vi "Parse Arguments.vi"(8 "error in (no error)":errorcluster, 9 "Args":string[](array[string]), 10 "Folder":path, 11 "UpdateAction in":refnum<class "UpdateAction.lvclass">) -> (0 "error out":errorcluster, 3 "UpdateAction out":refnum<class "UpdateAction.lvclass">)   [LabVIEW 2020, in "GPackTools.lvlib" / "UpdateAction.lvclass"]
uses:
  UpdateAction.lvclass
  UpdateAction.lvclass/UpdateAction.ctl
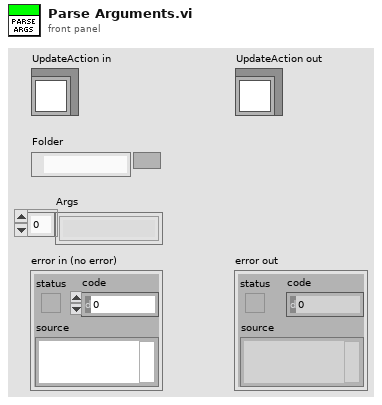
[diagram p1: front panel]
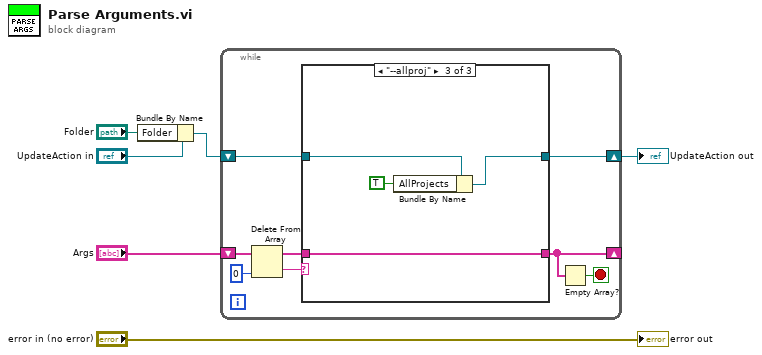
[diagram p0: block diagram]
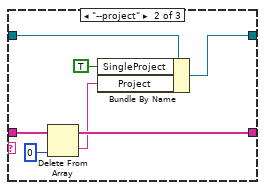
[diagram p3: hidden frame]
diagram:
  n1 = Bundle By Name(cluster="UpdateAction in", "Folder"="Folder") -> (w2:refnum<class "UpdateAction.lvclass">)
  n2 = while {
    shift-right: [w7] -> w3
    shift-left: w2 -> [w8]
    shift-right: [w10] -> _
    shift-left: "Args" -> [w14]
    stop <- w9 stop-if-true
    n3 = Delete From Array(array=w14, index=0) -> (deleted portion=w12:string, array with subset deleted=w11:string[])  [unwired: 1 in]
    n4 = case shown="\"--allproj\"" w12 {
      tunnel: w11 -> [w16 w22 w27]
      tunnel: [w16 w20 w27] -> w10
      tunnel: w8 -> [w15 w23 w26]
      tunnel: [w15 w19 w25] -> w7
      frame Default {
      }
      frame "--project" {
        n5 = Delete From Array(array=w22, index=0) -> (deleted portion=w18:string, array with subset deleted=w20:string[])  [unwired: 1 in]
        n6 = Bundle By Name(cluster=w23, "SingleProject"=TRUE, "Project"=w18) -> (w19:refnum<class "UpdateAction.lvclass">)
      }
      frame "--allproj" {
        n7 = Bundle By Name(cluster=w26, "AllProjects"=TRUE) -> (w25:refnum<class "UpdateAction.lvclass">)
      }
    }
    n8 = Empty Array?(array=w10) -> (empty?=w9:bool)
  }
  "UpdateAction out" <- w3
  "error out" <- "error in (no error)"
